vi "TSPopup.Show Popup.vi"(6 "Font Size":u32, 8 "error in (no error)":errorcluster, 9 "Call Data (ignore if empty)":variant, 10 "Popup Parameters":T1, 11 "TSPopup in":refnum<class "TSPopup.lvclass">) -> (0 "error out":errorcluster, 3 "TSPopup out":refnum<class "TSPopup.lvclass">)   [LabVIEW 2016, in "TSPopup.lvlib" / "TSPopup.lvclass"]
doc: "Invokes the Type Sensitive Popup using the provided Parameters. This <B>MUST</B> be used in the 'Mouse Down<B>?</B>' event, which is the filtering event. This makes the popup visible before allowing the mouse click to be handled.\n\n<B>Popup Parameters</B> - Parameters for showing the Type Sensitive Popup.\n<B>Call data</B> - This input will be returned with the 'Popup Event' for use in handling the Popup results.\n<B>Font Size</B> - If wired, this sets the font size of popups.\n\nType Sensitive Popup \nCopyright © 2007, J. David Saunders\nAll rights reserved."
uses:
  <userlib>/TSPopup/TSPopup.lvclass
  <userlib>/TSPopup/TSPopup.Popup Call Parameters.ctl
  <userlib>/TSPopup/TSPopup.Data Type.ctl
  <userlib>/TSPopup/TSPopup.lvclass/TSPopup.ctl
panel:
  # "Type Sensitive Popup \nCopyright © 2007, J. David Saunders\nAll rights reserved."
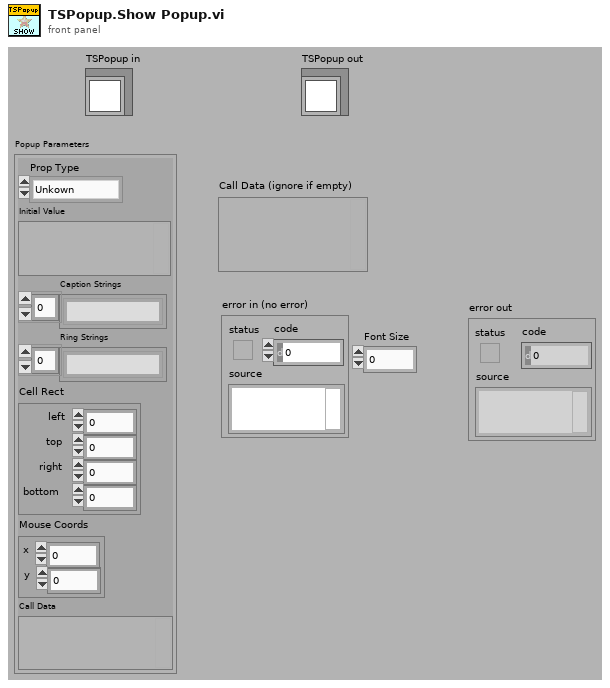
[diagram p1: front panel]
types:
  T1 = typedef "TSPopup.lvlib/TSPopup.lvclass/TSPopup.Popup Call Parameters.ctl" = cluster{"Prop Type":T2, "Initial Value":variant, "Caption Strings":string[], "Ring Strings":string[], "Cell Rect":cluster{"left":i16, "top":i16, "right":i16, "bottom":i16}, "Mouse Coords":cluster{"x":i16, "y":i16}, "Call Data":variant}
  T2 = typedef "TSPopup.lvlib/TSPopup.lvclass/TSPopup.Data Type.ctl" = enum16{"Unkown", "NO POPUP", "String", "Integer", "Float", "Color", "Boolean", "Ring", "Captioned String", "Captioned Integer", "Button Color", "2 Int Cluster", "4 Int Cluster", "check"}
  T3 = typedef "TSPopup.lvlib/TSPopup.lvclass/TSPopup.Monitor Register Data.ctl" = cluster{"Control":refnum<vi>, "Events":T4[]}
  T4 = typedef "TSPopup.lvlib/TSPopup.lvclass/TSPopup.Event Enum.ctl" = enum16{"Nothing", "Enter Key Accept", "Escape Key Cancel", "Mouse Outside Accept", "Mouse Outside Cancel", "Mouse Move Accept", "Mouse Move Cancel", "Mouse Leave Cancel", "Value Change Accept", "Lose Focus Cancel", "Cancel Button", "Accept Button"}
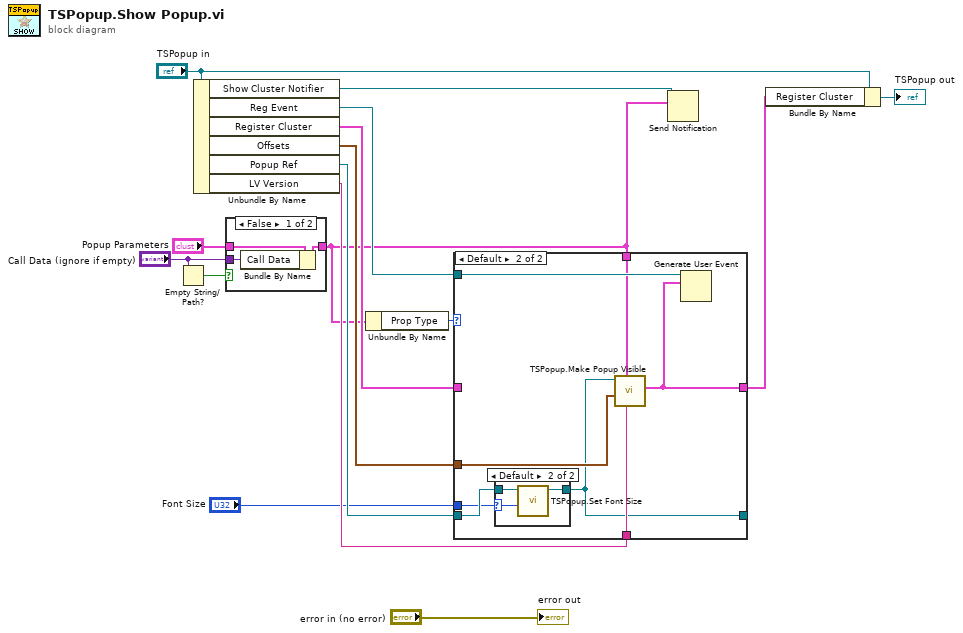
[diagram p0: block diagram]
diagram:
  n1 = Empty String/Path?(string/path="Call Data (ignore if empty)") -> (empty?=w15:bool)
  n2 = Unbundle By Name("TSPopup in") -> ("Show Cluster Notifier"=w2:refnum<notifier>, "Reg Event"=w10:refnum<user-event>, "Register Cluster"=w9:T3, "Offsets"=w8:cluster{"Left":i32, "Top":i32}[], "Popup Ref"=w7:refnum<vi>, "LV Version"=w6:string)
  n3 = case shown="False" w15 {
    tunnel: "Popup Parameters" -> [w18 w20]
    tunnel: "Call Data (ignore if empty)" -> [w19 _]
    tunnel: [w17 w20] -> w1
    frame False {
      n4 = Bundle By Name(cluster=w18, "Call Data"=w19) -> (w17:T1)
    }
    frame True {
    }
  }
  n5 = Unbundle By Name(w1) -> ("Prop Type"=w4:T2)
  n6 = case shown="Default" w4 {
    tunnel: w10 -> [_ w30]
    tunnel: w8 -> [_ w29]
    tunnel: [w22 w28] -> w5
    tunnel: w1 -> [_ w27]
    tunnel: w6 -> [_ w26]
    tunnel: w7 -> [w21 w25]
    tunnel: [w21 w24] -> _
    tunnel: w9 -> [w22 _]
    tunnel: "Font Size" -> [_ w23]
    frame "NO POPUP" {
    }
    frame Default {
      n7 = case shown="Default" w23 {
        selector: w23 -> [_ w34]
        tunnel: w25 -> [w31 w33]
        tunnel: [w31 w32] -> w24
        frame 0 {
        }
        frame Default {
          n8 = call <userlib>:"TSPopup.Set Font Size.vi"("Font Size"=w34, "Popup Cluster Ref"=w33) -> ("dup ref out"=w32:refnum<vi>)  [unwired: 8 in, 1 out]
        }
      }
      n9 = call <userlib>:"TSPopup.Make Popup Visible.vi"("LV Version"=w26, "Popup Parameters"=w27, "Ctl Offsets"=w29, "Popup Cluster Ref"=w24) -> ("event data"=w28:T3)  [unwired: 6 in, 1 out]
      n10 = Generate User Event(user event=w30, event data cluster=w28) -> ()  [unwired: 2 in, 2 out]
    }
  }
  n11 = Send Notification(notification=w1, notifier=w2) -> ()  [unwired: 1 in, 2 out]
  n12 = Bundle By Name(cluster="TSPopup in", "Register Cluster"=w5) -> (→"TSPopup out":refnum<class "TSPopup.lvclass">)
  "error out" <- "error in (no error)"
